vi "增加一条测试类型3自动测试记录.vi"(8 "测试结果":string, 9 "测试项":string, 10 "输入通道":i32, 11 "输出通道":i32) -> ()   [LabVIEW 2010]
uses:
  全局量/自动测试结果.vi
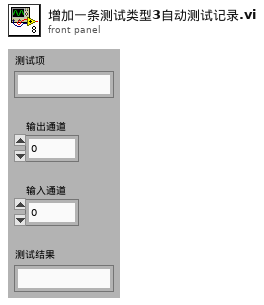
[diagram p1: front panel]
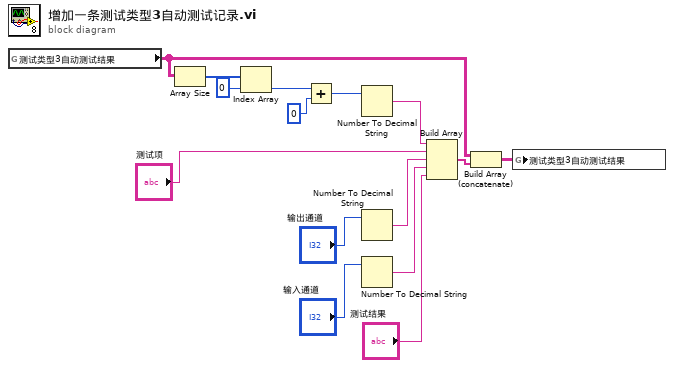
[diagram p0: block diagram]
diagram:
  n1 = global read "自动测试结果.vi" "测试类型3自动测试结果"() -> (w9:string[][])
  n2 = Array Size(array=w9) -> (size(s)=w15:i32[])
  n3 = Index Array(array=w15, index=0 ("索引")) -> (element=w13:i32)
  n4 = Add(x=w13, y=0) -> (x+y=w11:i32)
  n5 = Number To Decimal String(number=w11) -> (decimal integer string=w2:string)  [unwired: 1 in]
  n6 = Number To Decimal String(number="输出通道") -> (decimal integer string=w5:string)  [unwired: 1 in]
  n7 = Number To Decimal String(number="输入通道") -> (decimal integer string=w3:string)  [unwired: 1 in]
  n8 = Build Array(w2, "测试项", w5, w3, "测试结果") -> (w8:string[])
  n9 = Build Array (concatenate)(w9, w8) -> (w7:string[][])
  n10 = global write "自动测试结果.vi" "测试类型3自动测试结果"(w7) -> ()
